vi "setSpectTempSetpoint.vi"(8 "error in (no error)":errorcluster, 9 "command_setSpectTempSetpoint":T1, 10 "model in":refnum<class "IModel.lvclass">, 11 "NotImagingState in":refnum<class "NotImagingState.lvclass">) -> (0 "error out":errorcluster, 2 "model out":refnum<class "IModel.lvclass">, 3 "NotImagingState out":refnum<class "NotImagingState.lvclass">)   [LabVIEW 2016, in "States.lvlib" / "NotImagingState.lvclass"]
uses:
  NotImagingState.lvclass
  IModel/IModel.lvclass
  ts_sallv_sedspectrometer/DataTypes/command_setSpectTempSetpoint.ctl
  ts_sallv_sedspectrometer/SALLV_sedSpectrometer.lvlib
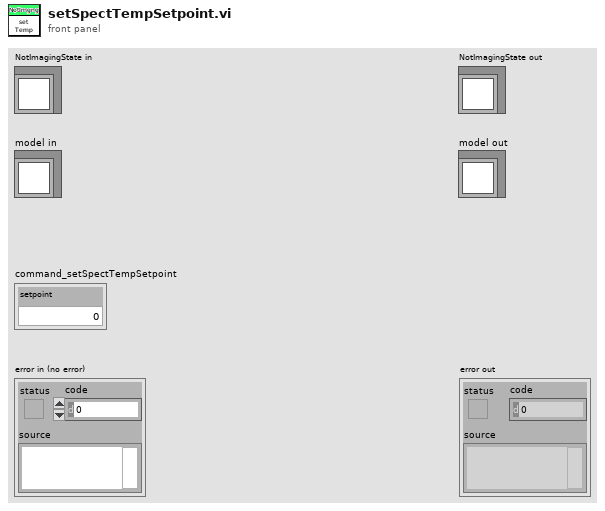
[diagram p1: front panel]
types:
  T1 = typedef "SALLV_sedSpectrometer.lvlib/command_setSpectTempSetpoint.ctl" = cluster{"setpoint":sgl}
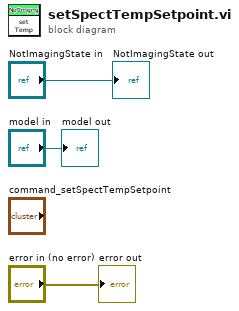
[diagram p0: block diagram]
diagram:
  "error out" <- "error in (no error)"
  "NotImagingState out" <- "NotImagingState in"
  "model out" <- "model in"
